vi "R7pHControl.vi"(8 "error constant":errorcluster, 11 "LabVIEW Web Service":refnum<class "Web Service.lvclass">) -> (0 "error out":errorcluster)   [LabVIEW 2016]
uses:
  <vilib>/wsapi/Web Service.lvclass
  Controls/pH_Manual Standard.ctl
  Controls/pH_SetParams Standard.ctl
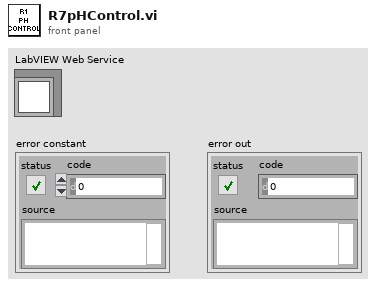
[diagram p1: front panel]
types:
  T1 = typedef "pH_Manual Standard.ctl" = cluster{"Acid Pump":bool, "Base Pump":bool}
  T2 = cluster{"Media Pump":bool, "Water Pump":bool, "Effluent Pump":bool, "Release Valve":bool, "N2 Valve":bool, "Recirc Pump":bool}
  T3 = typedef "pH_SetParams Standard.ctl" = cluster{"Set Point":dbl, "Tolerance":dbl, "Pump Time On, secs":dbl}
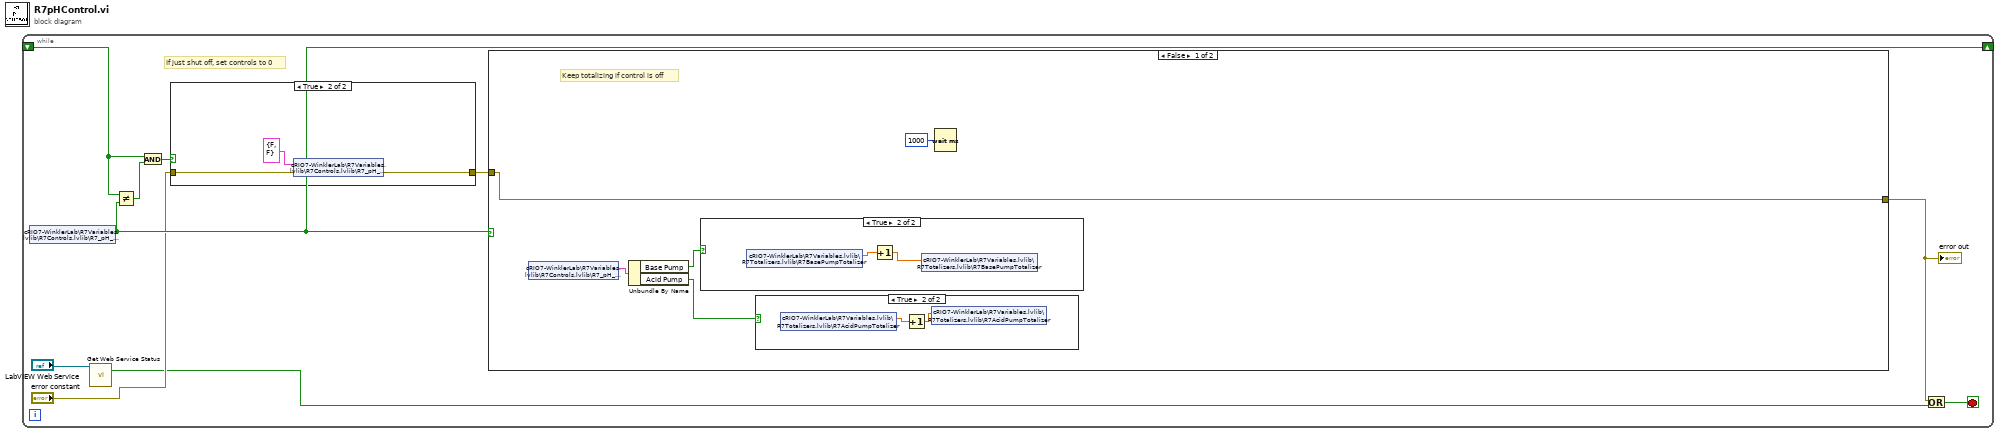
[diagram p0: block diagram]
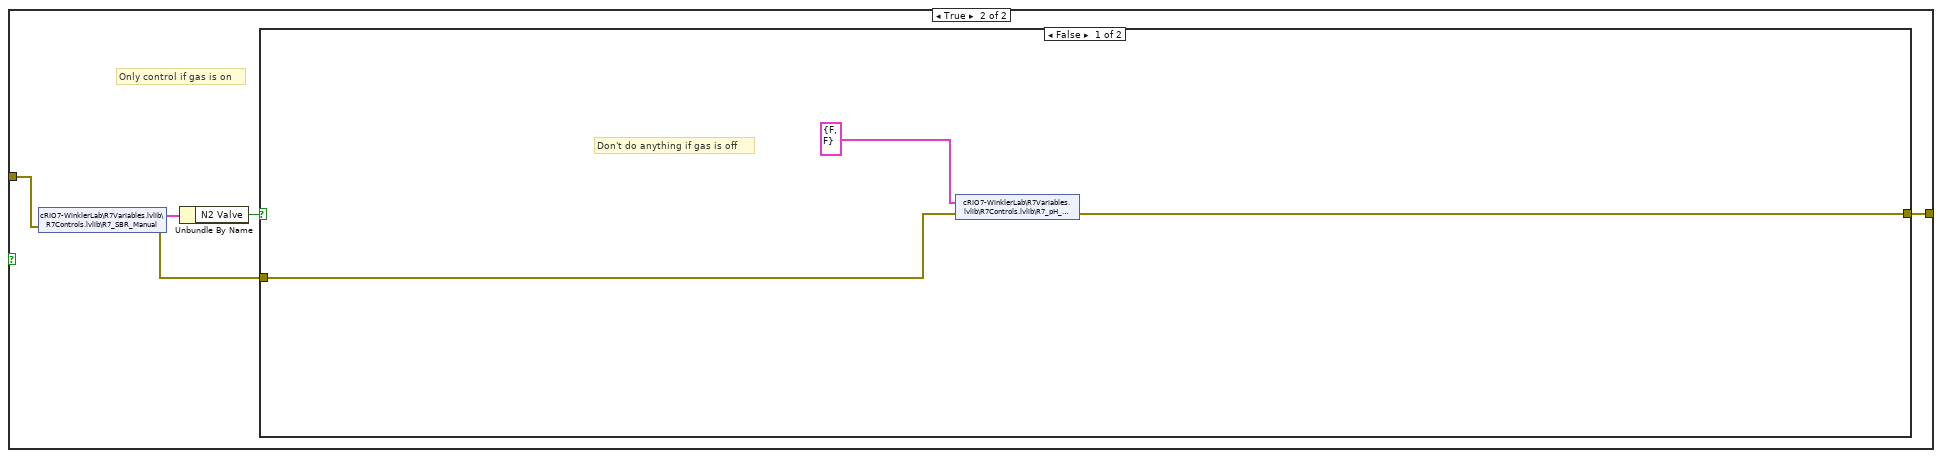
[diagram p5: hidden frame]
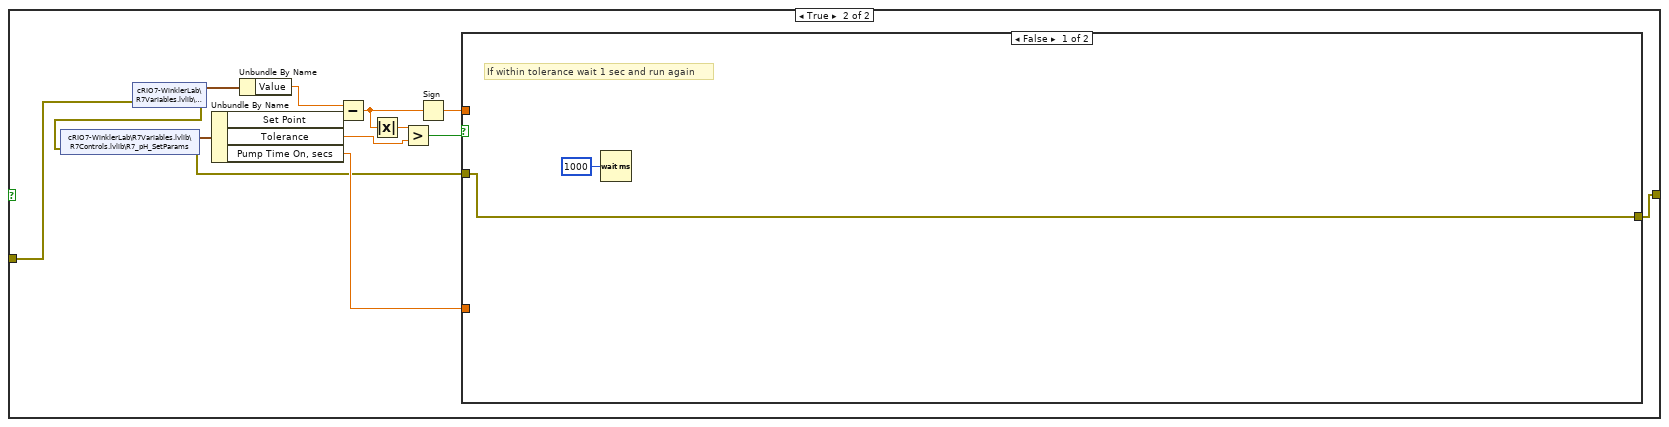
[diagram p6: hidden frame]
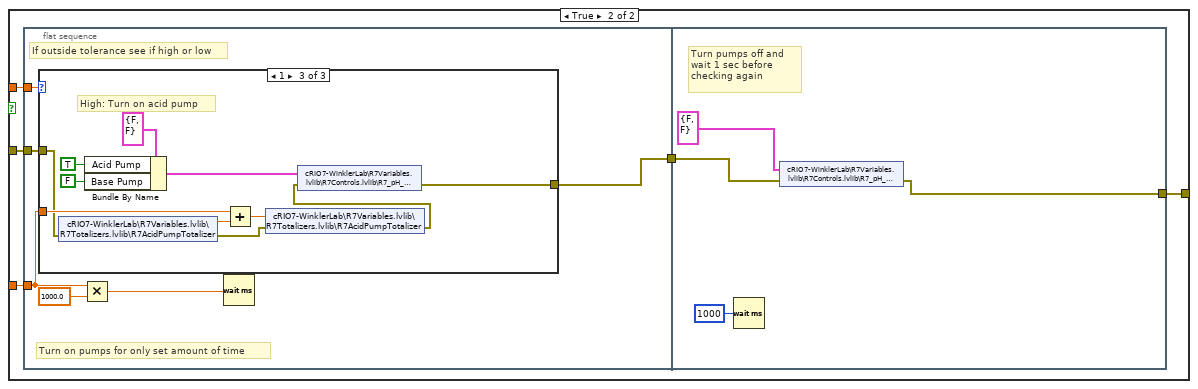
[diagram p7: hidden frame]
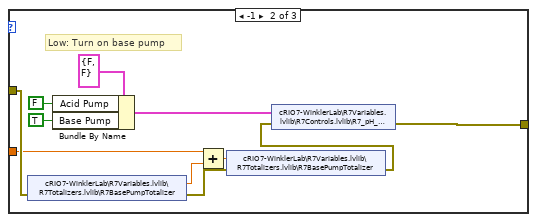
[diagram p9: hidden frame]
diagram:
  n1 = while {
    shift-right: [w8] -> _
    shift-left: _ -> [w7]
    stop <- w1 stop-if-true
    # "If just shut off, set controls to 0"
    n2 = shared-variable "cRIO7-WinklerLab\\R7Variables.lvlib\\R7Controls.lvlib\\R7_pH_Switch"() -> (w8:bool)  [unwired: 1 in, 1 out]
    n3 = call <vilib>:"Get Web Service Status.vi"("LabVIEW Web Service"="LabVIEW Web Service") -> ("service stopping?"=w3:bool)  [unwired: 12 in, 2 out]
    n4 = Not Equal?(x=w7, y=w8) -> (x != y?=w9:bool)
    n5 = And(x=w7, y=w9) -> (x .and. y?=w6:bool)
    n6 = case shown="True" w6 {
      tunnel: "error constant" -> [w11 w13]
      tunnel: [w11 w12] -> w4
      frame False {
      }
      frame True {
        n7 = shared-variable "cRIO7-WinklerLab\\R7Variables.lvlib\\R7Controls.lvlib\\R7_pH_Manual"(T1 {"Acid Pump"=FALSE, "Base Pump"=FALSE} ("R1pHManual"), error in=w13) -> (error out=w12:errorcluster)
      }
    }
    n8 = case shown="False" w8 {
      tunnel: w4 -> [w19 w26]
      tunnel: [w19 w24] -> w2
      frame False {
        # "Keep totalizing if control is off"
        n9 = shared-variable "cRIO7-WinklerLab\\R7Variables.lvlib\\R7Controls.lvlib\\R7_pH_Manual"() -> (w17:T1)  [unwired: 1 in, 1 out]
        n10 = Unbundle By Name(w17) -> ("Base Pump"=w16:bool, "Acid Pump"=w15:bool)
        n11 = case shown="True" w16 {
          frame False {
          }
          frame True {
            n12 = shared-variable "cRIO7-WinklerLab\\R7Variables.lvlib\\R7Totalizers.lvlib\\R7BasePumpTotalizer"() -> (w23:dbl)  [unwired: 1 in, 1 out]
            n13 = Increment(x=w23) -> (x+1=w22:dbl)
            n14 = shared-variable "cRIO7-WinklerLab\\R7Variables.lvlib\\R7Totalizers.lvlib\\R7BasePumpTotalizer"(w22) -> ()  [unwired: 1 in, 1 out]
          }
        }
        n15 = case shown="True" w15 {
          frame False {
          }
          frame True {
            n16 = shared-variable "cRIO7-WinklerLab\\R7Variables.lvlib\\R7Totalizers.lvlib\\R7AcidPumpTotalizer"() -> (w21:dbl)  [unwired: 1 in, 1 out]
            n17 = Increment(x=w21) -> (x+1=w20:dbl)
            n18 = shared-variable "cRIO7-WinklerLab\\R7Variables.lvlib\\R7Totalizers.lvlib\\R7AcidPumpTotalizer"(w20) -> ()  [unwired: 1 in, 1 out]
          }
        }
        n19 = Wait (ms)(milliseconds to wait=u32 1000) -> ()  [unwired: 1 out]
      }
      frame True {
        # "Only control if gas is on"
        n20 = shared-variable "cRIO7-WinklerLab\\R7Variables.lvlib\\R7Controls.lvlib\\R7_SBR_Manual"(error in=w26) -> (w27:T2, error out=w25:errorcluster)
        n21 = Unbundle By Name(w27) -> ("N2 Valve"=w28:bool)
        n22 = case shown="False" w28 {
          tunnel: w25 -> [w31 w35]
          tunnel: [w29 w32] -> w24
          frame False {
            # "Don't do anything if gas is off"
            n23 = shared-variable "cRIO7-WinklerLab\\R7Variables.lvlib\\R7Controls.lvlib\\R7_pH_Manual"(T1 {"Acid Pump"=FALSE, "Base Pump"=FALSE} ("R1pHManual"), error in=w31) -> (error out=w29:errorcluster)
          }
          frame True {
            n24 = shared-variable "cRIO7-WinklerLab\\R7Variables.lvlib\\R7Signals.lvlib\\R7pH"(error in=w35) -> (w45:cluster{"Signal":dbl, "Value":dbl}, error out=w34:errorcluster)
            n25 = shared-variable "cRIO7-WinklerLab\\R7Variables.lvlib\\R7Controls.lvlib\\R7_pH_SetParams"(error in=w34) -> (w44:T3, error out=w33:errorcluster)
            n26 = Unbundle By Name(w44) -> ("Set Point"=w42:dbl, "Tolerance"=w40:dbl, "Pump Time On, secs"=w36:dbl)
            n27 = Unbundle By Name(w45) -> ("Value"=w43:dbl)
            n28 = Subtract(x=w43, y=w42) -> (x-y=w38:dbl)
            n29 = Absolute Value(x=w38) -> (abs(x)=w41:dbl)
            n30 = Greater?(x=w41, y=w40) -> (0:w39:bool)
            n31 = Sign(1:w38) -> (0:w37:dbl)
            n32 = case shown="False" w39 {
              tunnel: w37 -> [_ w52]
              tunnel: w36 -> [_ w51]
              tunnel: w33 -> [w46 w50]
              tunnel: [w46 w48] -> w32
              frame False {
                # "If within tolerance wait 1 sec and run again"
                n33 = Wait (ms)(milliseconds to wait=u32 1000) -> ()  [unwired: 1 out]
              }
              frame True {
                n34 = flat-sequence {
                  tunnel: w52 -> [w58]
                  tunnel: w51 -> [w55]
                  tunnel: w50 -> [w54]
                  tunnel: [w53] -> w49
                  tunnel: w49 -> [w84]
                  tunnel: [w83] -> w48
                  frame #0 {
                    # "Turn on pumps for only set amount of time"
                    # "If outside tolerance see if high or low"
                    n35 = case shown="1" w58 {
                      tunnel: w55 -> [_ w60 w79]
                      tunnel: w54 -> [w59 w65 w75]
                      tunnel: [w59 w61 w71] -> w53
                      frame 0, Default {
                        # "Unless tolerance is 0 this code\nshouldn't be accesible"
                      }
                      frame -1 {
                        # "Low: Turn on base pump"
                        n36 = shared-variable "cRIO7-WinklerLab\\R7Variables.lvlib\\R7Totalizers.lvlib\\R7BasePumpTotalizer"(error in=w65) -> (w68:dbl, error out=w64:errorcluster)
                        n37 = Bundle By Name(cluster=T1 {"Acid Pump"=FALSE, "Base Pump"=FALSE} ("R1pHManual"), "Acid Pump"=FALSE, "Base Pump"=TRUE) -> (w63:T1)
                        n38 = Add(x=w60, y=w68) -> (x+y=w67:dbl)
                        n39 = shared-variable "cRIO7-WinklerLab\\R7Variables.lvlib\\R7Totalizers.lvlib\\R7BasePumpTotalizer"(w67, error in=w64) -> (error out=w62:errorcluster)
                        n40 = shared-variable "cRIO7-WinklerLab\\R7Variables.lvlib\\R7Controls.lvlib\\R7_pH_Manual"(w63, error in=w62) -> (error out=w61:errorcluster)
                      }
                      frame 1 {
                        # "High: Turn on acid pump"
                        n41 = shared-variable "cRIO7-WinklerLab\\R7Variables.lvlib\\R7Totalizers.lvlib\\R7AcidPumpTotalizer"(error in=w75) -> (w78:dbl, error out=w74:errorcluster)
                        n42 = Bundle By Name(cluster=T1 {"Acid Pump"=FALSE, "Base Pump"=FALSE} ("R1pHManual"), "Acid Pump"=TRUE, "Base Pump"=FALSE) -> (w73:T1)
                        n43 = Add(x=w79, y=w78) -> (x+y=w77:dbl)
                        n44 = shared-variable "cRIO7-WinklerLab\\R7Variables.lvlib\\R7Totalizers.lvlib\\R7AcidPumpTotalizer"(w77, error in=w74) -> (error out=w72:errorcluster)
                        n45 = shared-variable "cRIO7-WinklerLab\\R7Variables.lvlib\\R7Controls.lvlib\\R7_pH_Manual"(w73, error in=w72) -> (error out=w71:errorcluster)
                      }
                    }
                    n46 = Multiply(x=w55, y=1000.0) -> (x*y=w56:dbl)
                    n47 = Wait (ms)(milliseconds to wait=w56) -> ()  [unwired: 1 out]
                  }
                  frame #1 {
                    # "Turn pumps off and \nwait 1 sec before\nchecking again"
                    n48 = Wait (ms)(milliseconds to wait=u32 1000) -> ()  [unwired: 1 out]
                    n49 = shared-variable "cRIO7-WinklerLab\\R7Variables.lvlib\\R7Controls.lvlib\\R7_pH_Manual"(T1 {"Acid Pump"=FALSE, "Base Pump"=FALSE} ("R1pHManual"), error in=w84) -> (error out=w83:errorcluster)
                  }
                }
              }
            }
          }
        }
      }
    }
    "error out" <- w2
    n50 = Or(x=w2, y=w3) -> (x .or. y?=w1:bool)
  }
